vi "ErrorDataForDB.vi"(8 "error in (no error)":errorcluster, 11 "process error message":variant) -> (0 "error out":errorcluster, 3 "ErrorMessage":T1)   [LabVIEW 2015, in "CopyUtility.lvlib"]
uses:
  CopyUtility.lvlib
  controls/ErrorMessgae.ctl
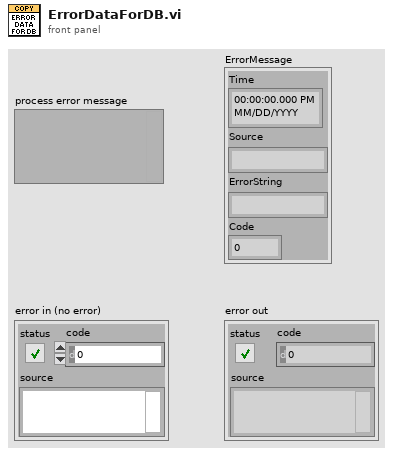
[diagram p1: front panel]
types:
  T1 = typedef "CopyUtility.lvlib/ErrorMessgae.ctl" = cluster{"Time":timestamp, "Source":string, "ErrorString":string, "Code":i32}
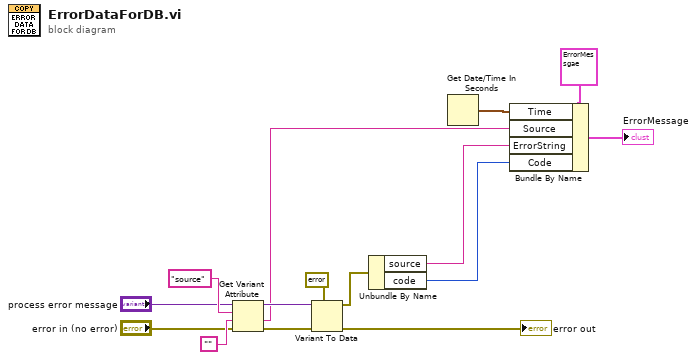
[diagram p0: block diagram]
diagram:
  n1 = Get Variant Attribute(Variant="process error message", name="source", default value (empty Variant)="", error in="error in (no error)") -> (duplicate Variant=w12:variant, value=w5:string, error out=w13:errorcluster)  [unwired: 1 out]
  n2 = Variant To Data(error in=w13, type=errorcluster {"status"=FALSE, "code"=0, "source"=""} ("error out"), Variant=w12) -> (data=w10:errorcluster, error out=→"error out":errorcluster)
  n3 = Unbundle By Name(w10) -> ("source"=w2:string, "code"=w1:i32)
  n4 = Get Date/Time In Seconds() -> (seconds since 1Jan1904=w4:timestamp)
  n5 = Bundle By Name(cluster=T1 {"Time"=timestamp(0 s since 1904-01-01), "Source"="", "ErrorString"="", "Code"=0} ("ErrorMessage"), "Time"=w4, "Source"=w5, "ErrorString"=w2, "Code"=w1) -> (→"ErrorMessage":T1)
